vi "Offset_comp_v1(SubVI).vi"(9 "DMARS Euler i":dbl[](array[numeric]), 10 "s":bool, 11 "Sim Euler Angle":dbl[](array[numeric])) -> (3 "Y_i":dbl[](array[numeric]))   [LabVIEW 2011]
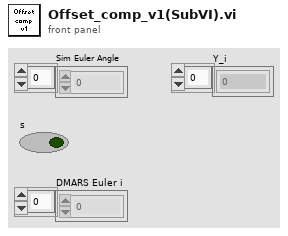
[diagram p1: front panel]
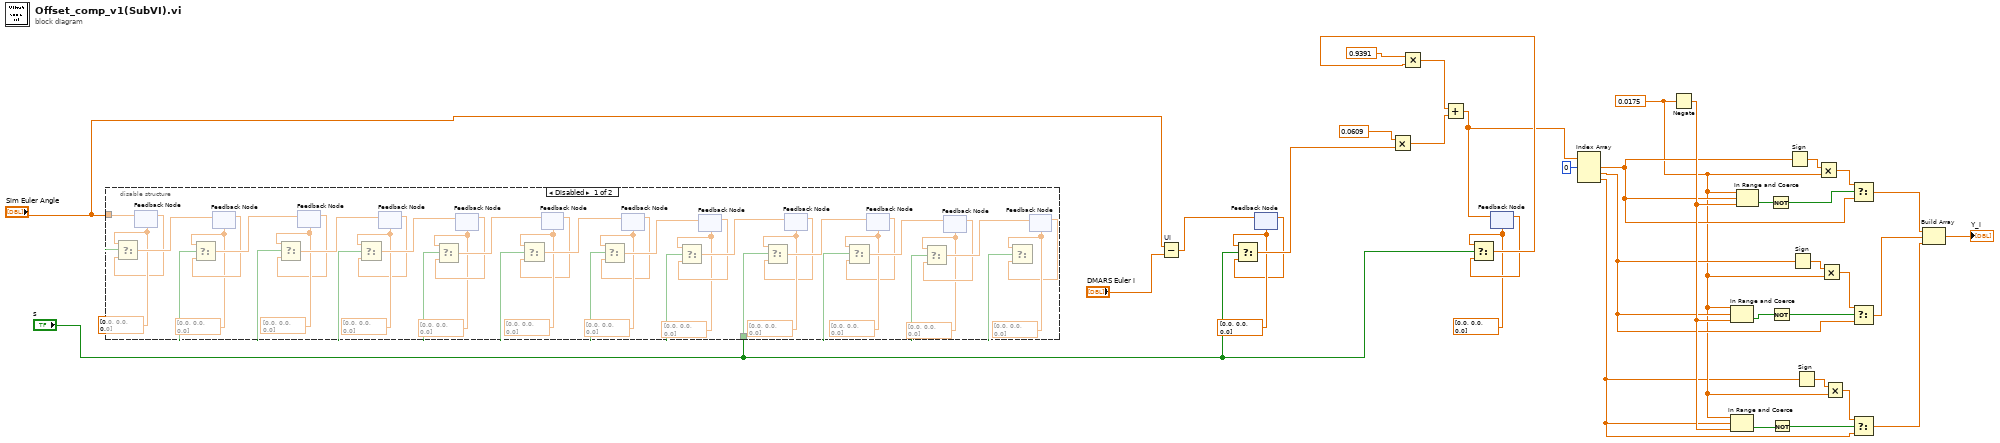
[diagram p0: block diagram]
diagram:
  w7 = 0.0175 ("upper limit")
  w26 = dbl[] [0.0, 0.0, 0.0] ("TVA_cmd")
  w28 = dbl[] [0.0, 0.0, 0.0] ("TVA_cmd")
  n1 = disable-structure shown="Disabled" {
    disable-tunnel: "s" -> [w74 _]
    disable-tunnel: "Sim Euler Angle" -> [w38 _]
    frame Disabled {
      w57 = dbl[] [0.0, 0.0, 0.0] ("TVA_cmd")
      w52 = dbl[] [0.0, 0.0, 0.0] ("TVA_cmd")
      w49 = dbl[] [0.0, 0.0, 0.0] ("TVA_cmd")
      w48 = dbl[] [0.0, 0.0, 0.0] ("TVA_cmd")
      w44 = dbl[] [0.0, 0.0, 0.0] ("TVA_cmd")
      w41 = dbl[] [0.0, 0.0, 0.0] ("TVA_cmd")
      w40 = dbl[] [0.0, 0.0, 0.0] ("TVA_cmd")
      w70 = dbl[] [0.0, 0.0, 0.0] ("TVA_cmd")
      w67 = dbl[] [0.0, 0.0, 0.0] ("TVA_cmd")
      w66 = dbl[] [0.0, 0.0, 0.0] ("TVA_cmd")
      w61 = dbl[] [0.0, 0.0, 0.0] ("TVA_cmd")
      w58 = dbl[] [0.0, 0.0, 0.0] ("TVA_cmd")
      n2 = feedback #1(w40) -> (w39:dbl[])
      n3 = Select(t=w40, s=w74, f=w39) -> (s? t:f=w45:dbl[])
      n4 = feedback-in #1(w38) -> ()
      n5 = feedback #2(w41) -> (w42:dbl[])
      n6 = Select(t=w41, s=w74, f=w42) -> (s? t:f=w46:dbl[])
      n7 = feedback-in #2(w45) -> ()
      n8 = feedback #3(w44) -> (w43:dbl[])
      n9 = Select(t=w44, s=w74, f=w43) -> (s? t:f=w55:dbl[])
      n10 = feedback-in #3(w46) -> ()
      n11 = feedback #4(w48) -> (w47:dbl[])
      n12 = Select(t=w48, s=w74, f=w47) -> (s? t:f=w53:dbl[])
      n13 = feedback-in #4(w55) -> ()
      n14 = feedback #5(w49) -> (w50:dbl[])
      n15 = Select(t=w49, s=w74, f=w50) -> (s? t:f=w54:dbl[])
      n16 = feedback-in #5(w53) -> ()
      n17 = feedback #6(w52) -> (w51:dbl[])
      n18 = Select(t=w52, s=w74, f=w51) -> (s? t:f=w64:dbl[])
      n19 = feedback-in #6(w54) -> ()
      n20 = feedback #7(w57) -> (w56:dbl[])
      n21 = Select(t=w57, s=w74, f=w56) -> (s? t:f=w62:dbl[])
      n22 = feedback-in #7(w64) -> ()
      n23 = feedback #8(w58) -> (w59:dbl[])
      n24 = Select(t=w58, s=w74, f=w59) -> (s? t:f=w63:dbl[])
      n25 = feedback-in #8(w62) -> ()
      n26 = feedback #9(w61) -> (w60:dbl[])
      n27 = Select(t=w61, s=w74, f=w60) -> (s? t:f=w73:dbl[])
      n28 = feedback-in #9(w63) -> ()
      n29 = feedback #10(w66) -> (w65:dbl[])
      n30 = Select(t=w66, s=w74, f=w65) -> (s? t:f=w71:dbl[])
      n31 = feedback-in #10(w73) -> ()
      n32 = feedback #11(w67) -> (w68:dbl[])
      n33 = Select(t=w67, s=w74, f=w68) -> (s? t:f=w72:dbl[])
      n34 = feedback-in #11(w71) -> ()
      n35 = feedback #12(w70) -> (w69:dbl[])
      n36 = Select(t=w70, s=w74, f=w69) -> ()  [unwired: 1 out]
      n37 = feedback-in #12(w72) -> ()
    }
    frame Enabled {
    }
  }
  n38 = Subtract "Ui"(x="Sim Euler Angle", y="DMARS Euler i") -> (x-y=w30:dbl[])
  n39 = feedback #13(w28) -> (w27:dbl[])
  n40 = Select(t=w28, s="s", f=w27) -> (s? t:f=w32:dbl[])
  n41 = feedback-in #13(w30) -> ()
  n42 = Multiply(x=0.0609, y=w32) -> (x*y=w35:dbl[])
  n43 = feedback #14(w26) -> (w36:dbl[])
  n44 = Select(t=w26, s="s", f=w36) -> (s? t:f=w37:dbl[])
  n45 = Multiply(x=0.9391, y=w37) -> (x*y=w34:dbl[])
  n46 = Add(x=w34, y=w35) -> (x+y=w24:dbl[])
  n47 = feedback-in #14(w24) -> ()
  n48 = Index Array(array=w24, index #1=0 ("index")) -> (element #1=w16:dbl, element #2=w11:dbl, element #3=w6:dbl)  [unwired: 2 in]
  n49 = Negate(x=w7) -> (-x=w22:dbl)
  n50 = In Range and Coerce(upper limit=w7, x=w6, lower limit=w22) -> (In Range?=w19:bool)  [unwired: 1 out]
  n51 = In Range and Coerce(upper limit=w7, x=w11, lower limit=w22) -> (In Range?=w20:bool)  [unwired: 1 out]
  n52 = In Range and Coerce(upper limit=w7, x=w16, lower limit=w22) -> (In Range?=w21:bool)  [unwired: 1 out]
  n53 = Not(x=w21) -> (.not. x?=w18:bool)
  n54 = Not(x=w20) -> (.not. x?=w15:bool)
  n55 = Not(x=w19) -> (.not. x?=w9:bool)
  n56 = Sign(1:w16) -> (0:w17:dbl)
  n57 = Sign(1:w11) -> (0:w13:dbl)
  n58 = Sign(1:w6) -> (0:w10:dbl)
  n59 = Multiply(x=w17, y=w7) -> (x*y=w14:dbl)
  n60 = Multiply(x=w13, y=w7) -> (x*y=w12:dbl)
  n61 = Multiply(x=w10, y=w7) -> (x*y=w8:dbl)
  n62 = Select(t=w14, s=w18, f=w16) -> (s? t:f=w5:dbl)
  n63 = Select(t=w12, s=w15, f=w11) -> (s? t:f=w4:dbl)
  n64 = Select(t=w8, s=w9, f=w6) -> (s? t:f=w3:dbl)
  n65 = Build Array(w5, w4, w3) -> (→"Y_i":dbl[])
